vi "GV_DBeditReply.vi"(8 "error in (no error)":errorcluster, 9 "Started?":bool, 11 "Gviewer in":refnum<class "Gviewer.lvclass">) -> (0 "error out":errorcluster, 3 "Gviewer out":refnum<class "Gviewer.lvclass">)   [LabVIEW 2020, in "Sgraph_lib_V1.lvlib" / "Gviewer.lvclass"]
doc: "Andre Koelewijn, 18 aug 2021\n\nReply from Gserver if the DB editor was started.\nIf not, then this VI will open the only allowed instance of the DB editor application."
uses:
  Gviewer.lvclass
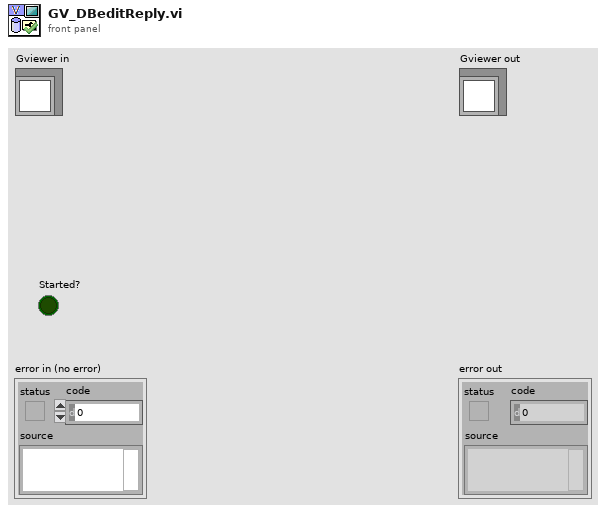
[diagram p1: front panel]
types:
  T1 = enum32{"Invalid", "Standard", "Closed", "Hidden", "Minimized", "Maximized"}
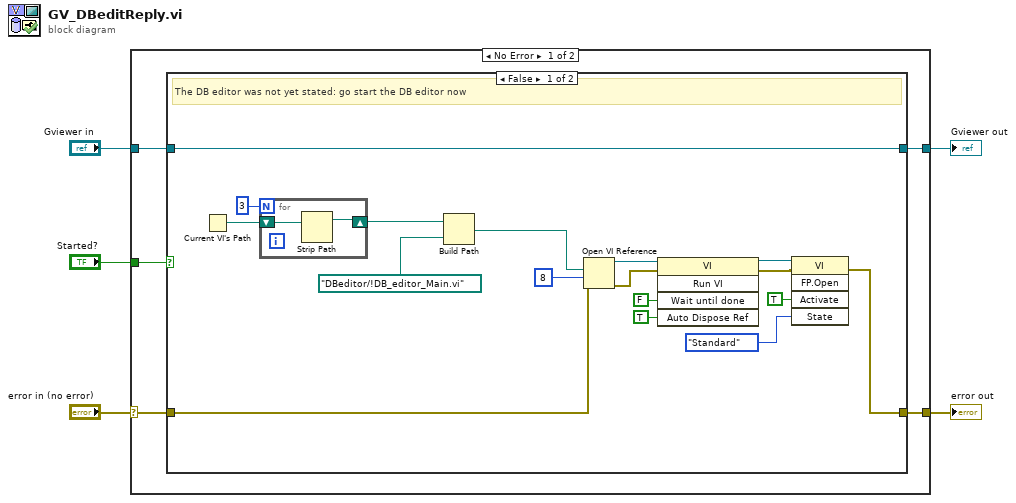
[diagram p0: block diagram]
diagram:
  n1 = case shown="No Error" "error in (no error)" {
    selector: "error in (no error)" -> [w8 w33]
    tunnel: [w7 w33] -> w4
    tunnel: [w6 w32] -> w2
    tunnel: "Gviewer in" -> [w9 w32]
    tunnel: "Started?" -> [w10 _]
    frame No Error {
      n2 = case shown="False" w10 {
        tunnel: w9 -> [w27 w30]
        tunnel: w8 -> [w20 w31]
        tunnel: [w13 w31] -> w7
        tunnel: [w27 w30] -> w6
        frame False {
          # "The DB editor was not yet stated: go start the DB editor now"
          n3 = Current VI's Path() -> (path=w26:path)
          n4 = for {
            N: 3 -> [_]
            shift-right: [w28] -> w24
            shift-left: w26 -> [w29]
            n5 = Strip Path(path=w29) -> (stripped path=w28:path)  [unwired: 1 out]
          }
          n6 = Build Path(base path=w24, name or relative path=path "DBeditor/!DB_editor_Main.vi") -> (appended path=w21:path)
          n7 = Open VI Reference(vi path=w21, options=8, error in (no error)=w20) -> (vi reference=w19:refnum<vi>, error out=w16:errorcluster)  [unwired: 3 in]
          n8 = invoke class="VI" method="Run VI"(reference=w19, error in=w16, "Wait until done"=FALSE ("Wait Until Done"), "Auto Dispose Ref"=TRUE ("Auto Dispose Reference")) -> (reference out=w15:refnum<vi>, error out=w14:errorcluster)  [unwired: 1 in, 3 out]
          n9 = invoke class="VI" method="FP.Open"(reference=w15, error in=w14, "Activate"=TRUE ("Activate?"), "State"=T1."Standard") -> (error out=w13:errorcluster)  [unwired: 1 in, 4 out]
        }
        frame True {
          # "The DB editor was already started: do nothing"
        }
      }
    }
    frame Error {
    }
  }
  "error out" <- w4
  "Gviewer out" <- w2
